vi "getChannelList.vi"(4 "error in (no error)":errorcluster, 5 "channel names":string, 6 "group name":string, 7 "tdms file":refnum<k34>) -> (0 "error out":errorcluster, 1 "channel names out":string[](array[string]), 2 "group names out":string[](array[string]), 3 "tdms file out":refnum<k34>)   [LabVIEW 2018]
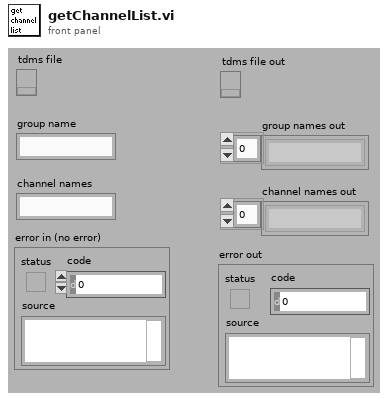
[diagram p1: front panel]
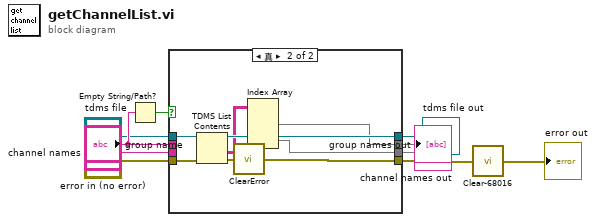
[diagram p0: block diagram]
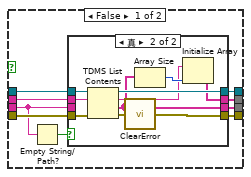
[diagram p2: hidden frame]
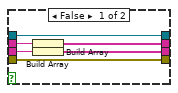
[diagram p3: hidden frame]
diagram:
  n1 = Empty String/Path?(string/path="group name") -> (empty?=w8:bool)
  n2 = case shown="真" w8 {
    tunnel: "tdms file" -> [w18 w43]
    tunnel: "error in (no error)" -> [w17 w42]
    tunnel: "channel names" -> [w16 _]
    tunnel: [w15 w40] -> w2
    tunnel: [w14 w41] -> w6
    tunnel: [w13 w39] -> w7
    tunnel: "group name" -> [w12 _]
    tunnel: [w11 w38] -> w10
    frame False {
      n3 = Empty String/Path?(string/path=w16) -> (empty?=w19:bool)
      n4 = case shown="真" w19 {
        tunnel: w18 -> [w24 w35]
        tunnel: w17 -> [w25 w34]
        tunnel: [w25 w33] -> w15
        tunnel: [w24 w32] -> w14
        tunnel: w12 -> [w21 w31]
        tunnel: [w22 w27] -> w13
        tunnel: w16 -> [w23 _]
        tunnel: [w20 w28] -> w11
        frame False {
          n5 = Build Array(w21) -> (w20:string[])
          n6 = Build Array(w23) -> (w22:string[])
        }
        frame True {
          n7 = TDMS List Contents(4:w34, 6:w31, 7:w35) -> (0:w26:errorcluster, 1:w27:string[], 2:w29:string, 3:w32:refnum<k34>)
          n8 = call "ClearError.vi"("error in (no error)"=w26) -> ("error out"=w33:errorcluster)
          n9 = Array Size(array=w27) -> (size(s)=w30:i32)
          n10 = Initialize Array(w29, w30) -> (w28:string[])
        }
      }
    }
    frame True {
      n11 = TDMS List Contents(4:w42, 7:w43) -> (0:w36:errorcluster, 1:w37:string[][], 3:w41:refnum<k34>)  [unwired: 1 in, 1 out]
      n12 = call "ClearError.vi"("error in (no error)"=w36) -> ("error out"=w40:errorcluster)
      n13 = Index Array(array=w37) -> (element #1=w38:string[], element #2=w39:string[])  [unwired: 4 in]
    }
  }
  "group names out" <- w10
  "channel names out" <- w7
  "tdms file out" <- w6
  n14 = call "Clear-68016.vi"("error in (no error)"=w2) -> ("error out"=→"error out":errorcluster)
